vi "MALT132 do you live.vi"() -> ()   [LabVIEW 2018]
uses:
  <instrlib>/AltonTech MALT/Public/Types/MALT Family Codes.ctl
  <instrlib>/AltonTech MALT/AltonTech MALT200817.lvlib
panel:
  in  "Address":i32=3 format="%02x"
  out "Live Status":bool
  in  "stop":bool
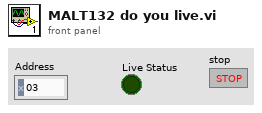
[diagram p1: front panel]
types:
  T1 = typedef "AltonTech MALT200817.lvlib/MALT Family Codes.ctl" = enum32{"-", "MALT40IO", "YAV904X8", "MALT132", "YAV91616", "MALT16PIN", "YAV90096", "YAV90HVT", "YAV90CLR", "YAV90128", "YAV90PNE", "MALTCON", "YAV91775", "YAV90XXX", "YAV90MMU", "H730050", "H710060", "H710061", "YAV90304", "MMI", "YAV90060", "MALT160T", "YAV90059", "Not Defined"}
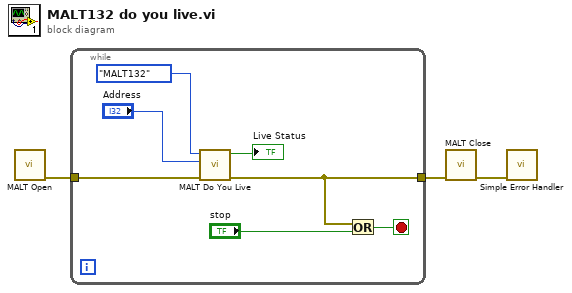
[diagram p0: block diagram]
diagram:
  n1 = call <instrlib>:"MALT Open.vi"() -> ("error out"=w3:errorcluster)  [unwired: 10 in, 1 out]
  n2 = while {
    tunnel: w3 -> [w8]
    tunnel: [w7] -> w1
    stop <- w10 stop-if-true
    n3 = call <instrlib>:"MALT Do You Live.vi"("error in"=w8, "Address"="Address", "MALT FamilyCode"=MALT_Family_Codes."MALT132") -> ("error out"=w7:errorcluster, "Live Status"=→"Live Status":bool)  [unwired: 7 in]
    n4 = Or(x=w7, y="stop") -> (x .or. y?=w10:bool)
  }
  n5 = call <instrlib>:"MALT Close.vi"("error in"=w1) -> ("error out"=w2:errorcluster)  [unwired: 10 in]
  n6 = call <vilib>:"Simple Error Handler.vi"("error in (no error)"=w2) -> ()  [unwired: 4 in, 5 out]
